vi "Engine In - Sensor - Fuel Temp.vi"(10 "Loop Freq [Hz]":sgl, 11 "Fuel Temp Raw [Ohm]":sgl) -> (3 "Fuel Temp [C]":sgl)   [LabVIEW 2015, in "ECS-RT.lvlib"]
uses:
  ECS-RT.lvlib
  <vilib>/ptbypt/NI_PtbyPt.lvlib
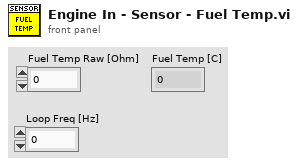
[diagram p1: front panel]
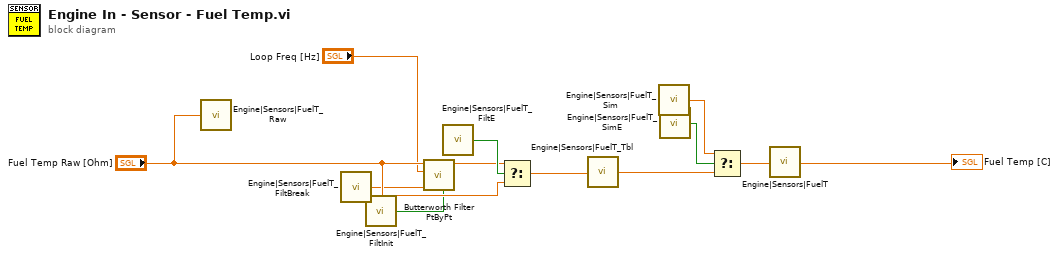
[diagram p0: block diagram]
diagram:
  n1 = call "Engine|Sensors|FuelT_Raw"("Value"="Fuel Temp Raw [Ohm]") -> ()
  n2 = call "Engine|Sensors|FuelT_FiltBreak"() -> ("Value"=w7:sgl)
  n3 = call "Engine|Sensors|FuelT_FiltInit"() -> ("Value"=w5:bool)
  n4 = call <vilib>:"Butterworth Filter PtByPt.vi"("initialize"=w5, "low cutoff freq: fl"=w7, "sampling freq: fs"="Loop Freq [Hz]", "x"="Fuel Temp Raw [Ohm]") -> ("Filtered x"=w6:dbl)  [unwired: 5 in, 1 out]
  n5 = call "Engine|Sensors|FuelT_FiltE"() -> ("Value"=w8:bool)
  n6 = Select(t=w6, s=w8, f="Fuel Temp Raw [Ohm]") -> (s? t:f=w3:dbl)
  n7 = call "Engine|Sensors|FuelT_Tbl"("X Index"=w3) -> ("Y"=w2:sgl)
  n8 = call "Engine|Sensors|FuelT_Sim"() -> ("Value"=w4:sgl)
  n9 = call "Engine|Sensors|FuelT_SimE"() -> ("Value"=w9:bool)
  n10 = Select(t=w4, s=w9, f=w2) -> (s? t:f=w11:sgl)
  "Fuel Temp [C]" <- w11
  n11 = call "Engine|Sensors|FuelT"("Value"=w11) -> ()
